vi "Configure Event Log.vi"(5 "Log Number (1: No 1)":i32(ring)=1 items=["No 1"=1, "No 2"=2, "No 3"=3, "No 4"=4], 6 "Log Message (\"\")":string, 7 "Log Level (0: Info)":i32(ring) items=["Info", "Warning", "Error"], 8 "error in (no error)":errorcluster, 10 "Block Number (0)":u32, 11 "VISA resource name":refnum<visa-resource-name>) -> (0 "error out":errorcluster, 3 "VISA resource name out":refnum<visa-resource-name>)   [LabVIEW 2016, in "Keithley DMM6500 DAQ6500 Series.lvlib"]
doc: "Allows you to log an event in the event log when the trigger model is running."
uses:
  Keithley DMM6500 DAQ6500 Series.lvlib
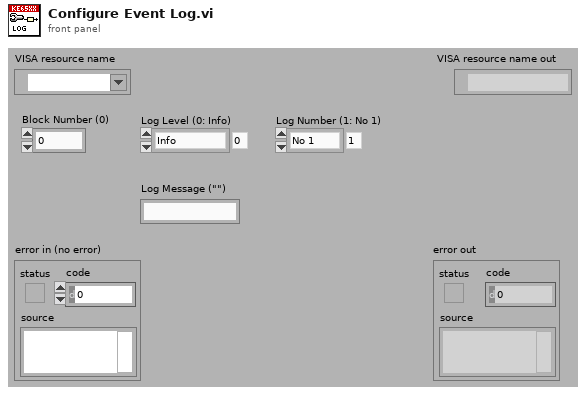
[diagram p1: front panel]
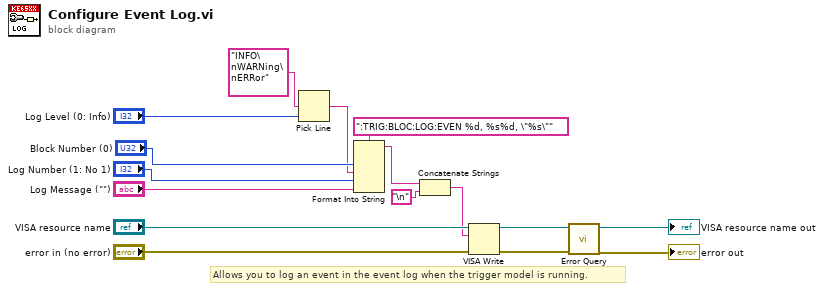
[diagram p0: block diagram]
diagram:
  # "Allows you to log an event in the event log when the trigger model is running."
  n1 = Pick Line(multi-line string="INFO\nWARNing\nERRor", line index="Log Level (0: Info)") -> (output string=w6:string)  [unwired: 1 in]
  n2 = Format Into String(format string=":TRIG:BLOC:LOG:EVEN %d, %s%d, \"%s\"", "Block Number (0)", w6, "Log Number (1: No 1)", "Log Message (\"\")") -> (resulting string=w2:string)  [unwired: 2 in, 1 out]
  n3 = Concatenate Strings(w2, "\n") -> (w3:string)
  n4 = VISA Write(VISA resource name="VISA resource name", write buffer=w3, error in (no error)="error in (no error)") -> (VISA resource name out=w10:refnum<visa-resource-name>, error out=w9:errorcluster)  [unwired: 1 out]
  n5 = call "Error Query.vi"("error in (no error)"=w9, "VISA resource name"=w10) -> ("error out"=→"error out":errorcluster, "VISA resource name out"=→"VISA resource name out":refnum<visa-resource-name>)  [unwired: 6 in, 2 out]
